vi "SetPersistentConfiguration.vi"(8 "ErrorIn":errorcluster, 9 "DataIn":variant, 11 "ObjectIn":refnum<class "ITAFObject.lvclass">) -> (0 "ErrorOut":errorcluster, 1 "DataOut":variant, 3 "ObjectOut":refnum<class "ITAFObject.lvclass">)   [LabVIEW 2021, in "ITAFObject.lvclass"]
uses:
  ITAFObject.lvclass
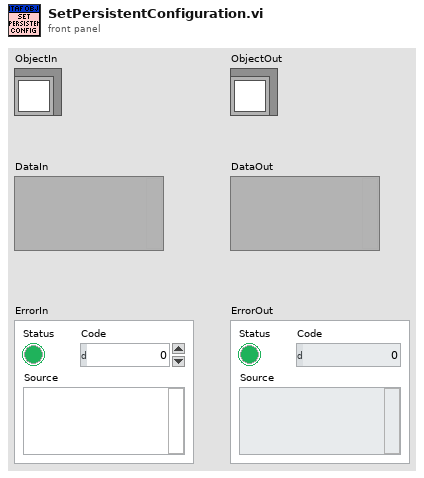
[diagram p1: front panel]
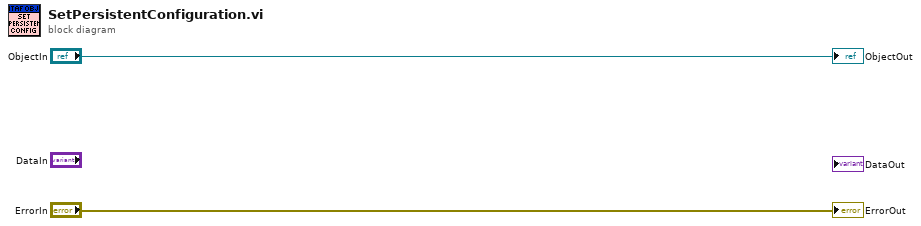
[diagram p0: block diagram]
diagram:
  "ErrorOut" <- "ErrorIn"
  "ObjectOut" <- "ObjectIn"
